vi "Find Child Aliases.vi"(7 "Actor in":refnum<class "Actor.lvclass">) -> (2 "Child Aliases":T1)   [LabVIEW 2020, in "jettl.lvlib" / "Actor Specific.lvlib"]
uses:
  Actor Specific.lvlib
  Actor/Actor.lvclass
  Child Aliases.ctl
  jettl.lvlib
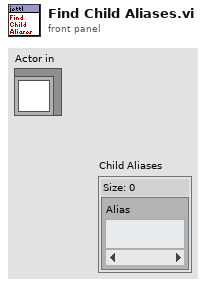
[diagram p1: front panel]
types:
  T1 = typedef "jettl.lvlib/Child Aliases.ctl" = set{string}
  T2 = typedef "jettl.lvlib/Child Attributes.ctl" = map{string, refnum<data-value>}
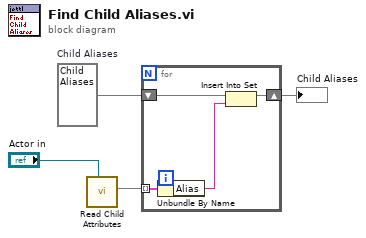
[diagram p0: block diagram]
diagram:
  w4 = T1 {}  # Child Aliases
  n1 = call "Read Child Attributes.vi"("Actor in"="Actor in") -> ("Child Attributes"=w1:T2)  [unwired: 10 in]
  n2 = for {
    shift-right: [w7] -> w3
    shift-left: w4 -> [w8]
    tunnel: w1 -> [w5] mode=indexing
    n3 = Unbundle By Name(w5) -> ("Alias"=w6:string)
    n4 = Insert Into Set(10:w6, 11:w8) -> (3:w7:T1)  [unwired: 1 out]
  }
  "Child Aliases" <- w3
